vi "SendOutputTrigger.vi"(8 "Error In":errorcluster, 10 "Output Trigger Configuration":T1={"Type"=enum."None", "Delay (ms)"=0, "Digital IO Line (1-14)"=1, "Digital IO Mode"=enum."Falling", "Digital IO Pulse Width (sec)"=0.0} {"Digital IO Line (1-14)" min=1 max=14 step=1}, 11 "Keithley 2602 In":refnum<visa-resource-name>) -> (0 "Error Out":errorcluster, 3 "Keithley 2602 Out":refnum<visa-resource-name>)   [LabVIEW 2012]
uses:
  TriggerOutputConfiguration.ctl
  TriggerOutputType.ctl
  driver/Public/Controls/TriggerMode.ctl
  driver/Keithley-2602.lvlib
  libs/LV-Utilities/LV-Utilities.lvlib
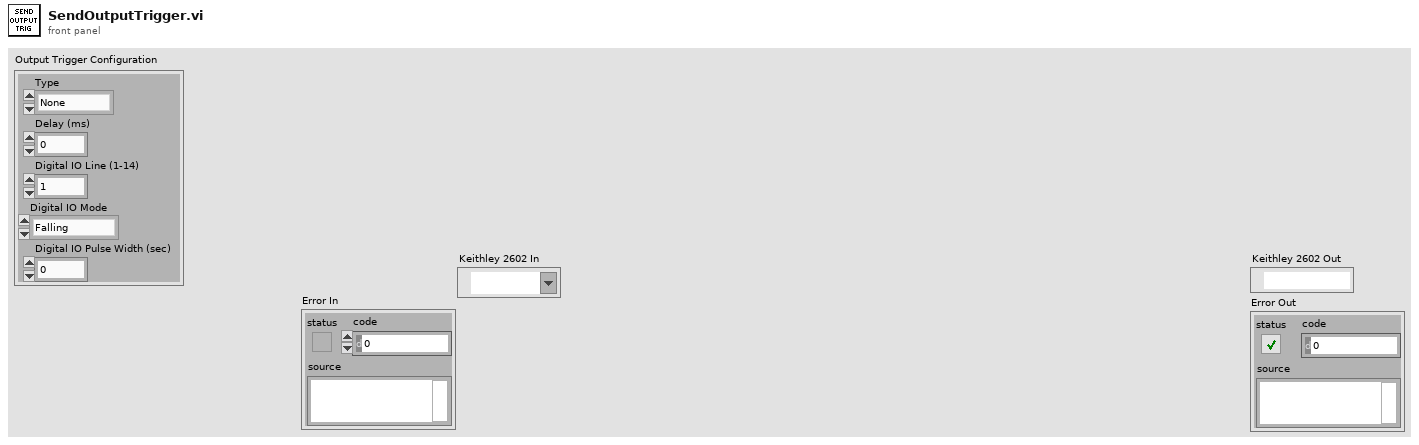
[diagram p1: front panel]
types:
  T1 = typedef "TriggerOutputConfiguration.ctl" = cluster{"Type":T2, "Delay (ms)":u32, "Digital IO Line (1-14)":u8, "Digital IO Mode":T3, "Digital IO Pulse Width (sec)":dbl}
  T2 = typedef "TriggerOutputType.ctl" = enum16{"None", "Digital IO", "Bus"}
  T3 = typedef "Keithley-2602.lvlib/TriggerMode.ctl" = enum16{"Falling", "Rising", "Either", "Synchronous"}
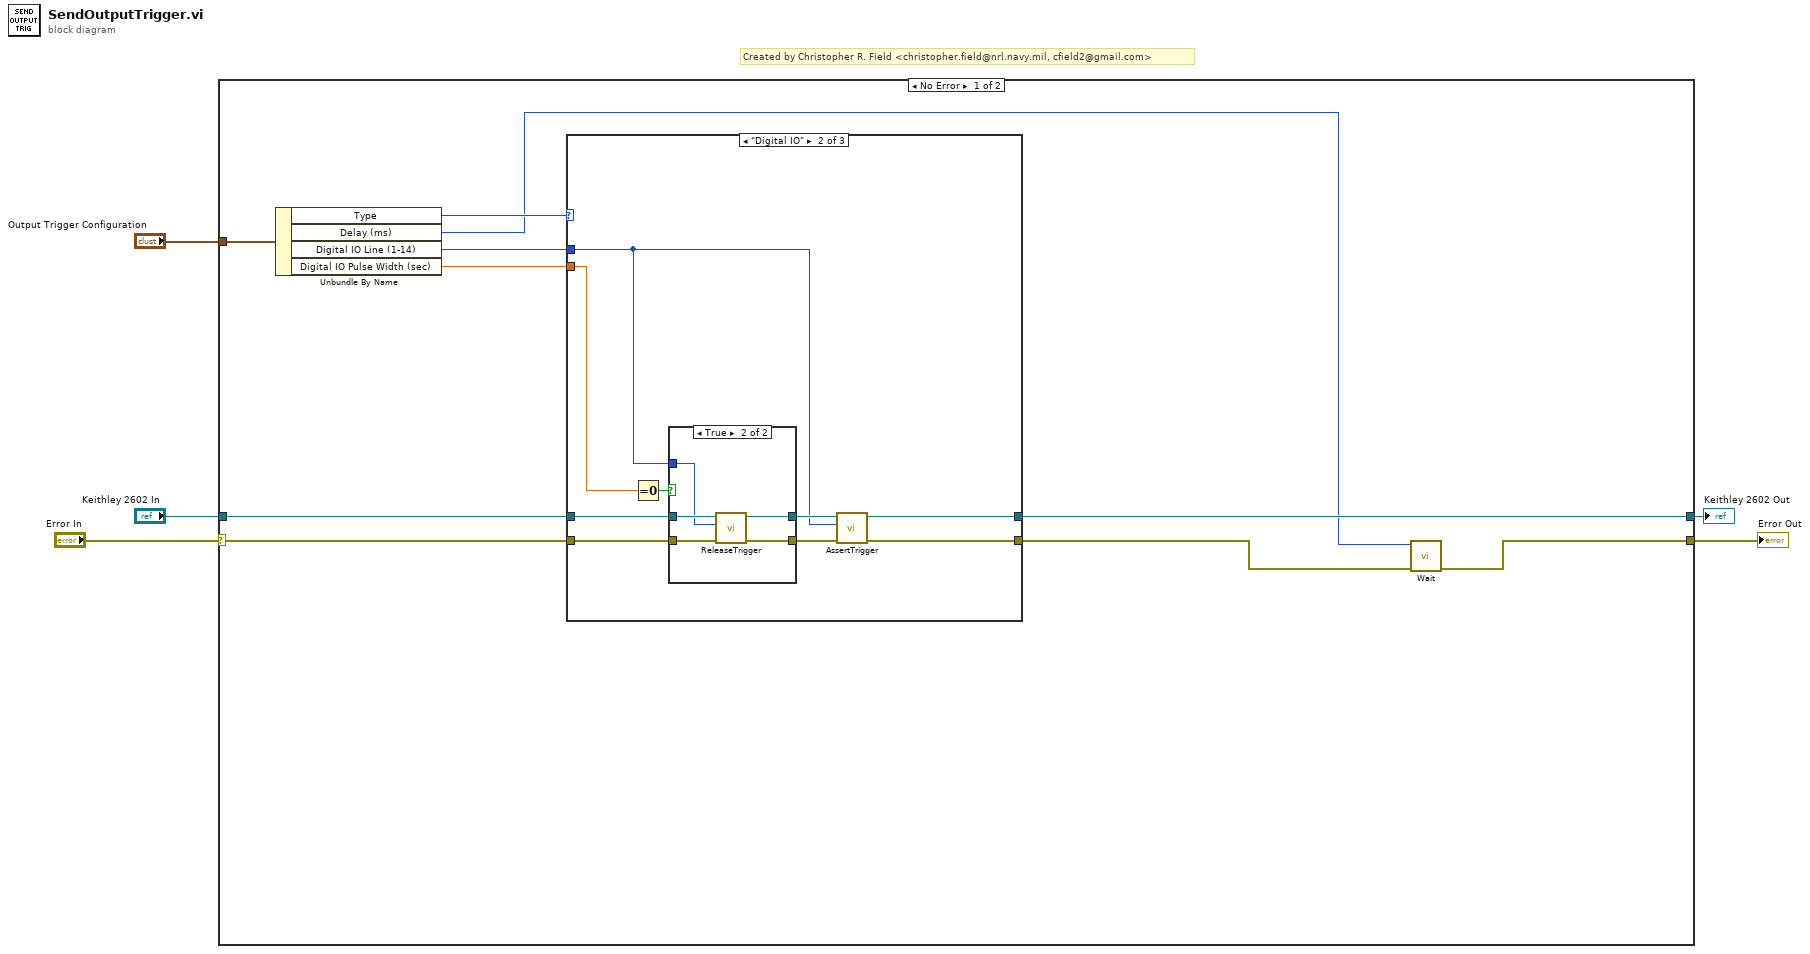
[diagram p0: block diagram]
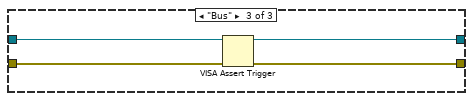
[diagram p4: hidden frame]
diagram:
  # "Created by Christopher R. Field <christopher.field@nrl.navy.mil, cfield2@gmail.com>"
  n1 = case shown="No Error" "Error In" {
    selector: "Error In" -> [w13 w38]
    tunnel: "Keithley 2602 In" -> [w15 w39]
    tunnel: [w14 w39] -> w3
    tunnel: [w11 w38] -> w2
    tunnel: "Output Trigger Configuration" -> [w10 _]
    frame No Error {
      n2 = Unbundle By Name(w10) -> ("Type"=w9:T2, "Delay (ms)"=w7:u32, "Digital IO Line (1-14)"=w8:u8, "Digital IO Pulse Width (sec)"=w6:dbl)
      n3 = case shown="\"Digital IO\"" w9 {
        tunnel: w15 -> [w17 w23 w37]
        tunnel: [w17 w26 w34] -> w14
        tunnel: w13 -> [w16 w19 w36]
        tunnel: [w16 w25 w35] -> w12
        tunnel: w8 -> [_ w18 _]
        tunnel: w6 -> [_ w24 _]
        frame "None", Default {
        }
        frame "Digital IO" {
          n4 = Equal To 0?(x=w24) -> (x = 0?=w22:bool)
          n5 = case shown="True" w22 {
            tunnel: w23 -> [w28 w33]
            tunnel: [w28 w32] -> w21
            tunnel: [w27 w31] -> w20
            tunnel: w19 -> [w27 w30]
            tunnel: w18 -> [_ w29]
            frame False {
            }
            frame True {
              n6 = call "ReleaseTrigger.vi"("Error In"=w30, "Line (1-14)"=w29, "Keithley 2602 In"=w33) -> ("Error Out"=w31:errorcluster, "Keithley 2602 Out"=w32:refnum<visa-resource-name>)  [unwired: 7 in]
            }
          }
          n7 = call "AssertTrigger.vi"("Error In"=w20, "Line (1-14)"=w18, "Keithley 2602 In"=w21) -> ("Error Out"=w25:errorcluster, "Keithley 2602 Out"=w26:refnum<visa-resource-name>)  [unwired: 7 in]
        }
        frame "Bus" {
          n8 = VISA Assert Trigger(8:w36, 11:w37) -> (0:w35:errorcluster, 3:w34:refnum<visa-resource-name>)  [unwired: 1 in]
        }
      }
      n9 = call "Wait.vi"("Error In"=w12, "Wait Time (msec)"=w7) -> ("Error Out"=w11:errorcluster)  [unwired: 9 in]
    }
    frame Error {
    }
  }
  "Keithley 2602 Out" <- w3
  "Error Out" <- w2
